vi "clusters and graphs.vi"() -> ()   [LabVIEW 2018]
panel:
  out "XY Graph":cluster{i32[], i32[]}(graph)
  in  "stop":bool
  out "Waveform Graph":i32[](graph)
  out "Waveform Chart":cluster{i32, i32}(graph)
  out "A3":cluster{"A2":bool, "A1":dbl, "A3":string}
  out "A2":cluster{"A2":bool, "A1":dbl, "A3":string}
  out "String":string
  out "Boolean":bool
  out "Numeric":dbl
  in  "A":cluster{"A2":bool, "A1":dbl, "A3":string}
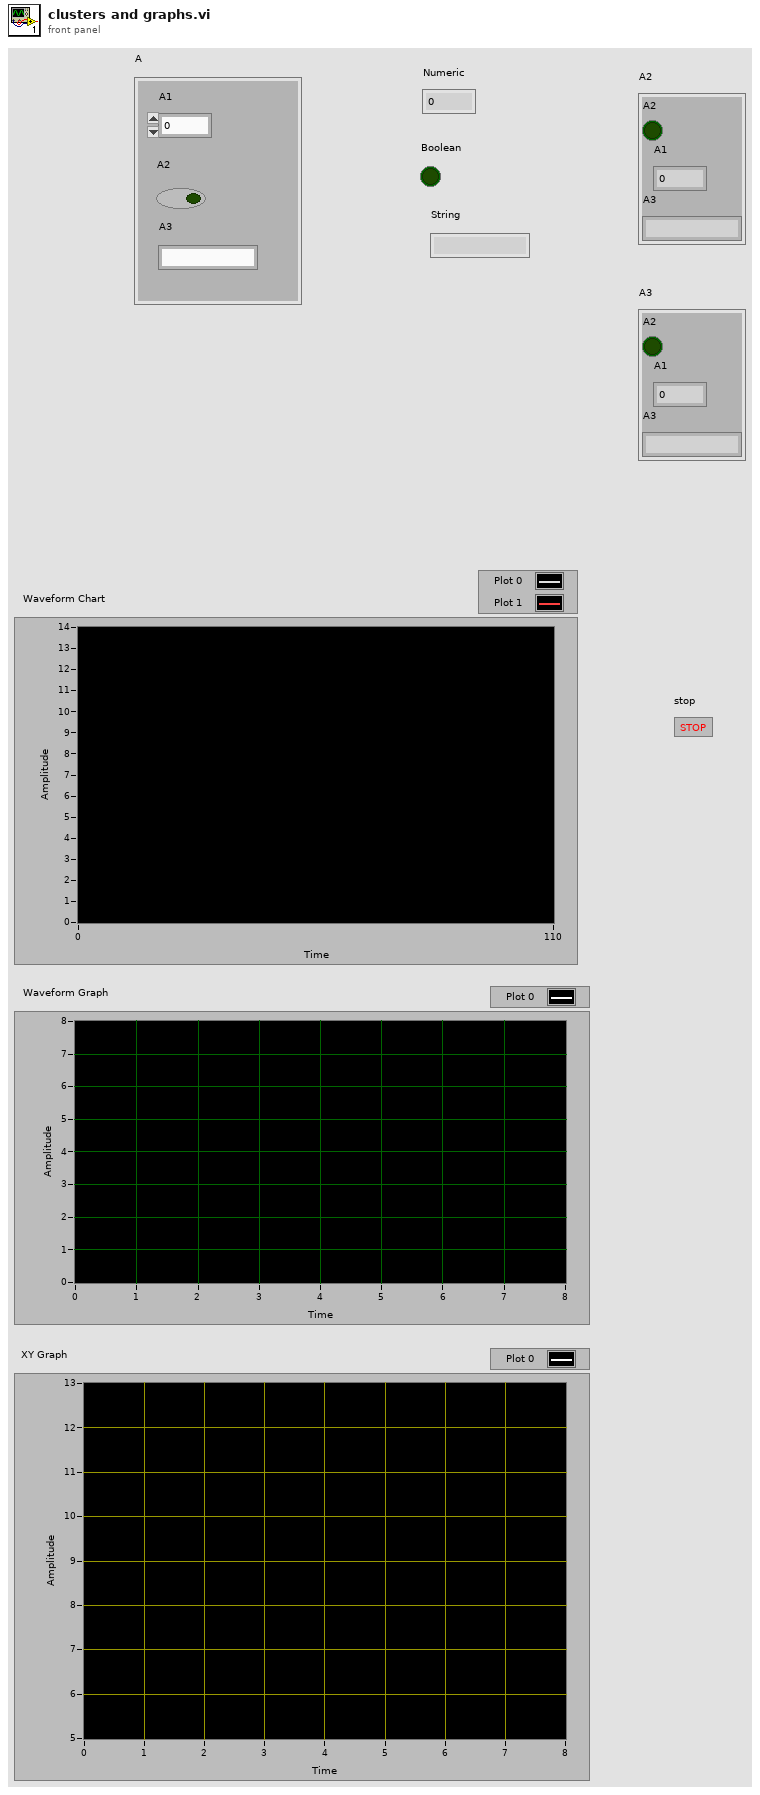
[diagram p1: front panel]
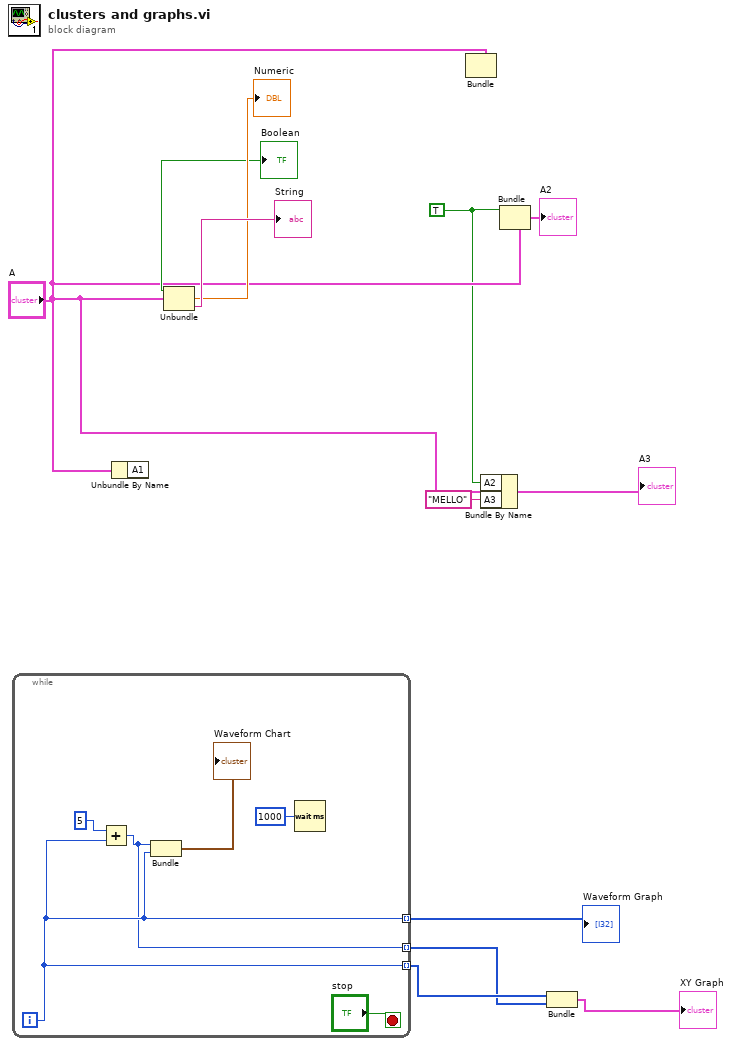
[diagram p0: block diagram]
diagram:
  w6 = TRUE ("A2")
  n1 = while {
    tunnel: [w14] -> w4 mode=indexing
    tunnel: [w14] -> w3 mode=indexing
    tunnel: [w13] -> w2 mode=indexing
    i -> [w14]
    stop <- "stop" stop-if-true
    n2 = Add(x=5, y=w14) -> (x+y=w13:i32)
    n3 = Bundle(w13, w14) -> (→"Waveform Chart":cluster{i32, i32})  [unwired: 1 in]
    n4 = Wait (ms)(milliseconds to wait=u32 1000) -> ()  [unwired: 1 out]
  }
  "Waveform Graph" <- w4
  n5 = Unbundle By Name("A") -> ()  [unwired: 1 out]
  n6 = Unbundle("A") -> ("A2"=→"Boolean":bool, "A1"=→"Numeric":dbl, "A3"=→"String":string)
  n7 = Bundle(cluster="A") -> ()  [unwired: 3 in, 1 out]
  n8 = Bundle By Name(cluster="A", "A2"=w6, "A3"="MELLO") -> (→"A3":cluster{"A2":bool, "A1":dbl, "A3":string})
  n9 = Bundle(cluster="A", "A2"=w6) -> (→"A2":cluster{"A2":bool, "A1":dbl, "A3":string})  [unwired: 2 in]
  n10 = Bundle(w3, w2) -> (→"XY Graph":cluster{i32[], i32[]})  [unwired: 1 in]
